vi "Testbench.vi"() -> ()   [LabVIEW 2015]
uses:
  <vilib>/FPGAPlugInAG/sbRIO-9607/niLvFpga_Open_sbRIO-9607.vi
  <vilib>/rvi/interface/common/dynamic/niFpgaDynamicAddResources.vi
  <vilib>/Utility/error.llb/Error Cluster From Error Code.vi
  <vilib>/rvi/errors/niLvFpgaAdjustHostInterfaceError.vi
  <vilib>/FPGAPlugInAG/Dynamic/niLvFpga_Close_Dynamic.vi
  <vilib>/rvi/interface/nirviOpenFPGA/nirviOpenFPGA.xnode
  FPGA Bitfiles/SVPWMdev_FPGATarget_SVPWMTestHarness_7zYtsrE0qaU.lvbitx
  SVPWMTestHarness.vi
  <vilib>/rvi/interface/nirviReadWriteControl/nirviReadWriteControl.xnode
  <vilib>/rvi/interface/nirviCloseFPGA/nirviCloseFPGA.xnode
  SVPWMInterface/SVPWMInterface.lvlib
  <vilib>/rvi/DesktopExecutionNode/DesktopExecutionNode.xnode
  <vilib>/rvi/DesktopExecutionNode/Execution/niFpgaDEN_Execute.vi
  NiFpgaLv.dll
  <vilib>/rvi/interface/Simulation/niFpgaSimulationCallBeginRW.vi
panel:
  out "appended array":dbl[][](graph)
  in  "modulation":fxp<+/-,16,2>
  in  "engauge":bool
  in  "Deadtime":u8=5
  in  "Period":u32=4000
  out "SimSignals":sgl[][](graph)
  in  "FXP":bool
  out "position":i32
  out "velocity":i32
  out "acceleration":i32
  in  "enable":bool
  in  "freq":sgl=10.0
  in  "stop":bool
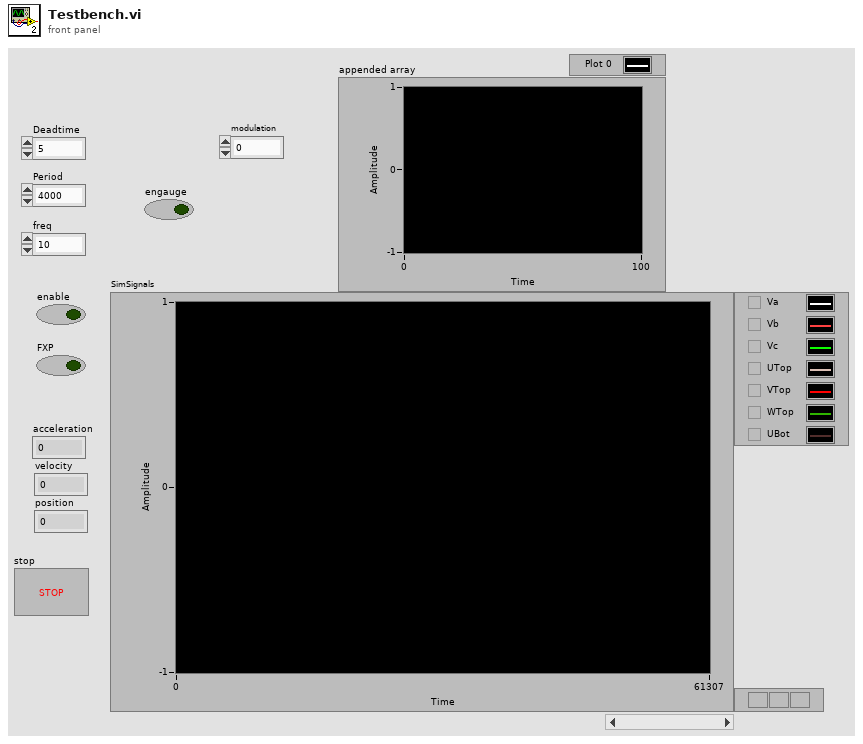
[diagram p1: front panel]
types:
  T1 = typedef "SVPWM.lvlib/SVPWM_SGL.ctl" = cluster{"max":sgl, "Period":u32, "Deadtime":u8}
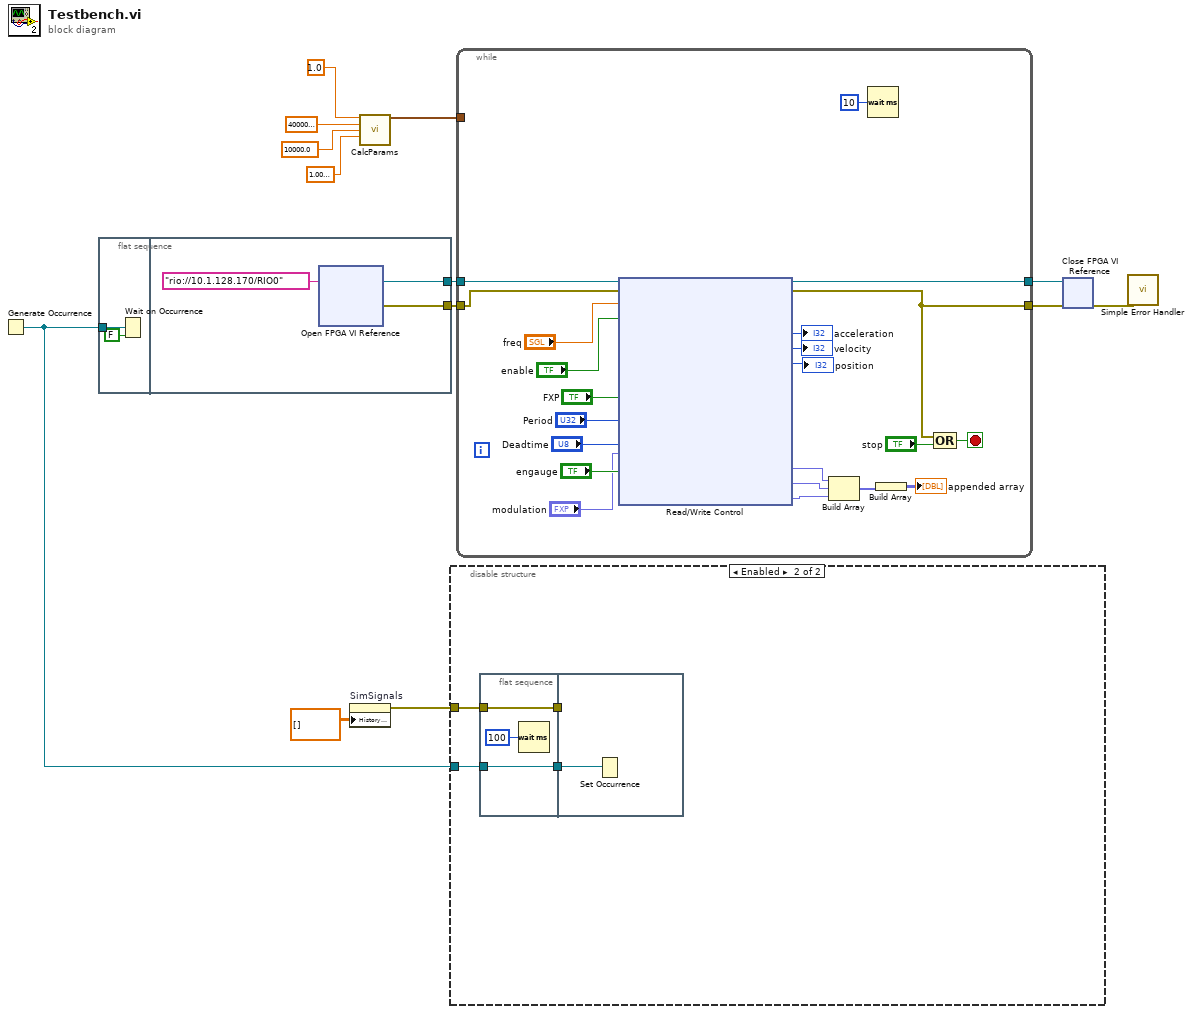
[diagram p0: block diagram]
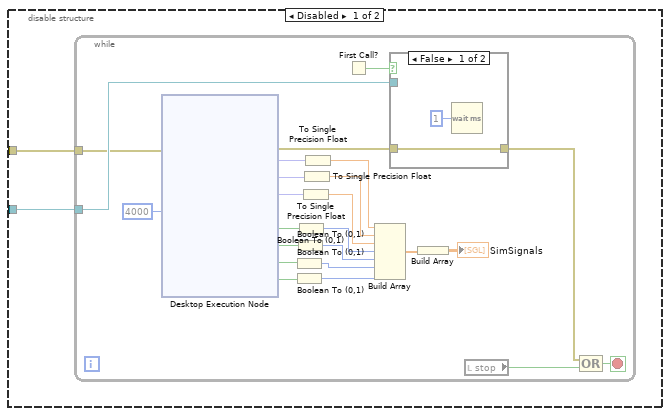
[diagram p2: hidden frame]
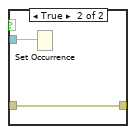
[diagram p3: hidden frame]
diagram:
  n1 = Generate Occurrence() -> (w6:refnum<k4>)
  n2 = flat-sequence {
    tunnel: w6 -> [w15]
    tunnel: [w18] -> w13
    tunnel: [w16] -> w3
    frame #0 {
      n3 = Wait on Occurrence(1:FALSE ("ignore previous (T)"), 2:w15) -> ()  [unwired: 1 in, 1 out]
    }
    frame #1 {
      n4 = xnode "Open FPGA VI Reference"("resource name"=tag "rio://10.1.128.170/RIO0") -> ("FPGA VI Reference Out"=w18:refnum<k20>, "error out"=w16:errorcluster)  [unwired: 1 in]
    }
  }
  n5 = property on="SimSignals" class="WFChart (strict)"("History Data"=sgl[][] []) -> (error out=w4:errorcluster)  [unwired: 2 in, 1 out]
  n6 = call "CalcParams.vi"("Max"=sgl 1.0, "ClkRate"=sgl 40000000.0, "fc"=sgl 10000.0, "deadtime"=sgl 1e-07) -> ("Parameters"=w8:T1)  [unwired: 11 in]
  n7 = disable-structure shown="Enabled" {
    disable-tunnel: w6 -> [w20 w52]
    disable-tunnel: w4 -> [w19 w51]
    frame Disabled {
      n8 = while {
        tunnel: w20 -> [w44]
        tunnel: w19 -> [w24]
        stop <- w43 stop-if-true
        n9 = xnode "Desktop Execution Node"("Error In"=w24, "Period"=u32 4000) -> ("Error Out"=w23:errorcluster, "A"=w41:fxp<+/-,32,4>, "B"=w40:fxp<+/-,32,4>, "C"=w39:fxp<+/-,32,4>, "s2B / uTOPB"=w38:bool, "s4B / vTOPB"=w37:bool, "s6B / wTOPB"=w21:bool, "s1B / uBOTB"=w36:bool)
        n10 = Boolean To (0,1)(Boolean=w21) -> (0, 1=w30:i16)
        n11 = Boolean To (0,1)(Boolean=w36) -> (0, 1=w29:i16)
        n12 = Boolean To (0,1)(Boolean=w37) -> (0, 1=w31:i16)
        n13 = Boolean To (0,1)(Boolean=w38) -> (0, 1=w32:i16)
        n14 = To Single Precision Float(number=w39) -> (single precision float=w33:sgl)
        n15 = To Single Precision Float(number=w40) -> (single precision float=w34:sgl)
        n16 = To Single Precision Float(number=w41) -> (single precision float=w35:sgl)
        n17 = First Call?() -> (First Call?: T/F=w25:bool)
        n18 = Build Array(w35, w34, w33, w32, w31, w30, w29) -> (w28:sgl[])
        n19 = case shown="False" w25 {
          tunnel: w44 -> [_ w48]
          tunnel: w23 -> [w45 w47]
          tunnel: [w45 w47] -> w22
          frame False {
            n20 = Wait (ms)(milliseconds to wait=u32 1) -> ()  [unwired: 1 out]
          }
          frame True {
            n21 = Set Occurrence(w48) -> ()
          }
        }
        n22 = Build Array(w28) -> (→"SimSignals":sgl[][])
        n23 = local read "stop"() -> (w42:bool)
        n24 = Compound Arithmetic op=OR(w22, w42) -> (w43:bool)
      }
    }
    frame Enabled {
      n25 = flat-sequence {
        tunnel: w51 -> [w54]
        tunnel: w52 -> [w55]
        tunnel: [w55] -> w50
        tunnel: [w54] -> w49
        tunnel: w50 -> [w56]
        tunnel: w49 -> [_]
        frame #0 {
          n26 = Wait (ms)(milliseconds to wait=u32 100) -> ()  [unwired: 1 out]
        }
        frame #1 {
          n27 = Set Occurrence(w56) -> ()
        }
      }
    }
  }
  n28 = while {
    tunnel: w13 -> [w78]
    tunnel: w8 -> [_]
    tunnel: [w76] -> w7
    tunnel: w3 -> [w69]
    tunnel: [w66] -> w2
    stop <- w67 stop-if-true
    n29 = xnode "Read/Write Control"("FPGA VI Reference In"=w78, "error in"=w69, "freq"="freq", "enable"="enable", "FXP"="FXP", "Period"="Period", "Deadtime"="Deadtime", "engauge"="engauge", "modulation"="modulation") -> ("FPGA VI Reference Out"=w76:refnum<k20>, "error out"=w66:errorcluster, "acceleration (counts/interval^2)"=→"acceleration":i32, "velocity (counts/interval)"=→"velocity":i32, "position (counts)"=→"position":i32, "A"=w61:fxp<+/-,32,4>, "B"=w60:fxp<+/-,32,4>, "C"=w59:fxp<+/-,32,4>)  [unwired: 1 out]
    n30 = Build Array(w61, w60, w59) -> (w58:fxp<+/-,32,4>[])
    n31 = Wait (ms)(milliseconds to wait=u32 10) -> ()  [unwired: 1 out]
    n32 = Build Array(w58) -> (→"appended array":fxp<+/-,32,4>[][])
    n33 = Compound Arithmetic op=OR(w66, "stop") -> (w67:bool)
  }
  n34 = xnode "Close FPGA VI Reference"("FPGA VI Reference In"=w7, "error in"=w2) -> ("error out"=w1:errorcluster)
  n35 = call <vilib>:"Simple Error Handler.vi"("error in (no error)"=w1) -> ()  [unwired: 4 in, 5 out]
